vi "ISX3_Parse_SyncTime.vi"(0 "Array":u8[](array[numeric])) -> (1 "SyncTime in µs":u32)   [LabVIEW 2012, in "Sciospec ISX3 Impedance Analyzer.lvlib"]
uses:
  Sciospec ISX3 Impedance Analyzer.lvlib
panel:
  # "This VI parses a data frame that contains a sync time setting."
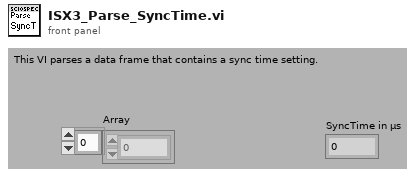
[diagram p1: front panel]
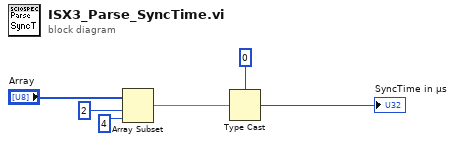
[diagram p0: block diagram]
diagram:
  n1 = Array Subset(array="Array", index=2 ("Index"), length=4 ("Länge")) -> (w5:u8[])
  n2 = Type Cast(type=u32 0, x=w5) -> (*(type *) &x=→"SyncTime in µs":u32)
